vi "Stash Framework.vi"(10 "Files and Folders":path[](array[path])) -> (0 "error out":errorcluster)   [LabVIEW 2020]
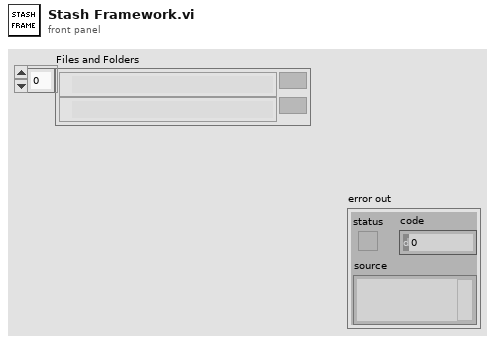
[diagram p1: front panel]
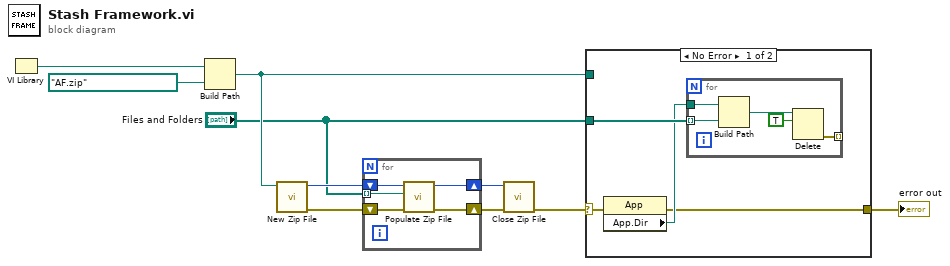
[diagram p0: block diagram]
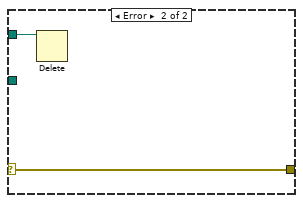
[diagram p2: hidden frame]
diagram:
  n1 = VI Library() -> (path=w9:path)
  n2 = Build Path(base path=w9, name or relative path=path "AF.zip") -> (appended path=w2:path)
  n3 = call <vilib>:"New Zip File.vi"("target"=w2) -> ("error out"=w7:errorcluster, "zip file out"=w8:i64)  [unwired: 2 in, 3 out]
  n4 = for {
    shift-right: [w14] -> w6
    shift-left: w7 -> [w15]
    tunnel: "Files and Folders" -> [w13] mode=indexing
    shift-right: [w12] -> w5
    shift-left: w8 -> [w11]
    n5 = call "Populate Zip File.vi"("error in (no error)"=w15, "Source"=w13, "zip file in"=w11) -> ("error out"=w14:errorcluster, "zip file out"=w12:i64)  [unwired: 7 in]
  }
  n6 = call <vilib>:"Close Zip File.vi"("error in (no error)"=w6, "zip file in"=w5) -> ("error out"=w4:errorcluster)  [unwired: 1 in, 4 out]
  n7 = case shown="No Error" w4 {
    selector: w4 -> [w19 w26]
    tunnel: [w16 w26] -> w3
    tunnel: w2 -> [_ w25]
    tunnel: "Files and Folders" -> [w18 _]
    frame No Error {
      n8 = property class="App"(error in=w19) -> (error out=w16:errorcluster, "App.Dir"=w17:path)  [unwired: 1 in, 1 out]
      n9 = for {
        tunnel: w18 -> [w24] mode=indexing
        tunnel: w17 -> [w22]
        tunnel: [w21] -> _ mode=indexing
        n10 = Build Path(base path=w22, name or relative path=w24) -> (appended path=w23:path)
        n11 = Delete(path (use dialog)=w23, entire hierarchy (F)=TRUE) -> (error out=w21:errorcluster)  [unwired: 3 in, 2 out]
      }
    }
    frame Error {
      n12 = Delete(path (use dialog)=w25) -> ()  [unwired: 4 in, 3 out]
    }
  }
  "error out" <- w3
